vi "Initialize Attributes.vi"(8 "error in (no error)":errorcluster, 10 "Attribute Data":variant, 11 "CS++MCS in":refnum<class "CS++MCS.lvclass">) -> (0 "error out":errorcluster, 2 "Found?":bool, 3 "CS++MCS out":refnum<class "CS++MCS.lvclass">)   [LabVIEW 2016, in "CS++MCS.lvlib" / "CS++MCS.lvclass"]
doc: "Initialize object attribute.\n\nUnique resources should be allocated elsewhere!"
uses:
  CS++MCS.lvclass
  C:/User/Brand/LVP/CSPP-Dev/Packages/CSPP_Core/Actors/CS++BaseActor/CS++BaseActor.lvclass
  PV-Enum.ctl
  CS++MCS.lvclass/CS++MCS.ctl
  CSPP_Core/Actors/CS++DeviceActor/CS++DeviceActor.lvclass
  CSPP_Core/Actors/CS++BaseActor/CS++BaseActor.lvclass
panel:
  in  "PV-Enum":T1
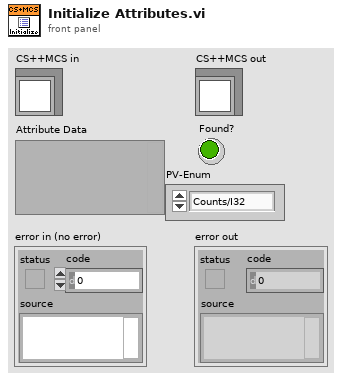
[diagram p1: front panel]
types:
  T1 = typedef "CS++MCS.lvlib/CS++MCS.lvclass/PV-Enum.ctl" = enum16{"Counts/I32", "TotalCounts/I32", "Status/I8", "BinWidth/Dbl", "NofBins/I32", "NofRecords /I32", "DiscLvl/Dbl", "TrigLvl/Dbl", "DiscSlope/U16", "TrigSlope/U16", "ActWaveform/AWfm|0:1"}
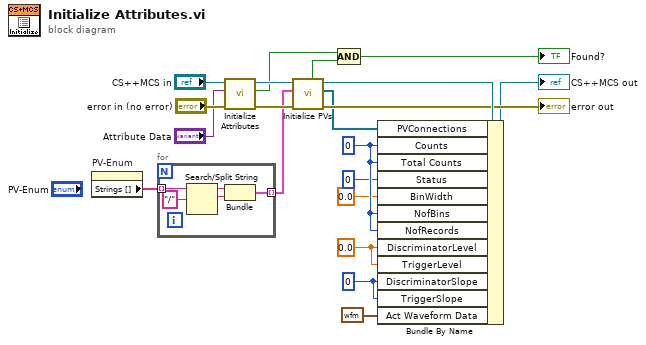
[diagram p0: block diagram]
diagram:
  w8 = dbl[unit] 0.0 ("DiscriminatorLevel")
  w10 = u16 0 ("DiscriminatorSlope")
  w12 = 0 ("Counts")
  n1 = property on="PV-Enum" class="Enum (strict)"() -> ("Strings []"=w4:string[])  [unwired: 2 in, 2 out]
  n2 = for {
    tunnel: w4 -> [w25] mode=indexing
    tunnel: [w21] -> w3 mode=indexing
    n3 = Search/Split String(string=w25, search string/char (-)="/") -> (substring before match=w23:string, match + rest of string=w22:string)  [unwired: 1 in, 1 out]
    n4 = Bundle(w23, w22) -> (w21:cluster{string, string})  [unwired: 1 in]
  }
  n5 = call-parent "Initialize Attributes.vi"("error in (no error)"="error in (no error)", "Attribute Data"="Attribute Data", "CS++DeviceActor in"="CS++MCS in") -> ("error out"=w15:errorcluster, "Found?"=w1:bool, "CS++DeviceActor out"=w17:refnum<class "CS++MCS.lvclass">)  [unwired: 6 in]
  n6 = call "Initialize PVs.vi"("error in (no error)"=w15, "SinglePVs"=w3, "CS++BaseActor in"=w17) -> ("error out"=→"error out":errorcluster, "PVConnections"=w5:refnum<class "PVConnection.lvclass">[], "CS++BaseActor out"=w16:refnum<class "CS++MCS.lvclass">, "Found?"=w2:bool)  [unwired: 4 in, 1 out]
  n7 = Compound Arithmetic op=AND(w1, w2) -> (→"Found?":bool)
  n8 = Bundle By Name(cluster=w16, "PVConnections"=w5, "Counts"=w12, "Total Counts"=w12, "Status"=i8 0, "BinWidth"=dbl[unit] 0.0, "NofBins"=w12, "NofRecords"=w12, "DiscriminatorLevel"=w8, "TriggerLevel"=w8, "DiscriminatorSlope"=w10, "TriggerSlope"=w10, "Act Waveform Data"=waveform(dbl) {"t0"=timestamp(0 s since 1904-01-01), "dt"=1.0, "Y"=[]}) -> (→"CS++MCS out":refnum<class "CS++MCS.lvclass">)
